vi "Build Filename.vi"(9 "Measurment Type":string, 11 "Metadata In":string[][](array[string])) -> (3 "String":string)   [LabVIEW 2014, in "Timing and Stabilization.lvlib"]
uses:
  Timing and Stabilization.lvlib
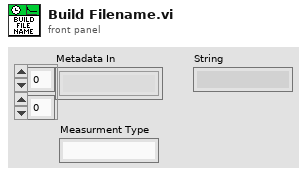
[diagram p1: front panel]
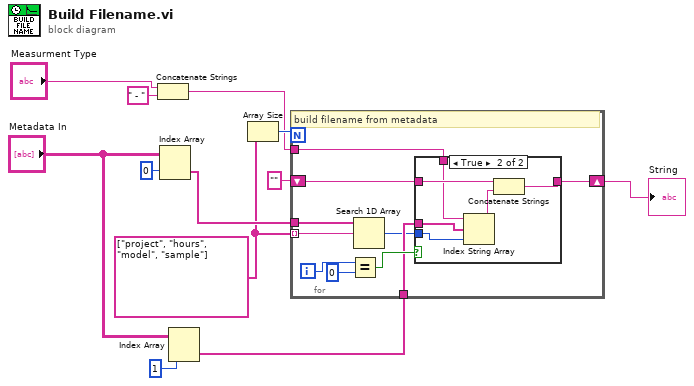
[diagram p0: block diagram]
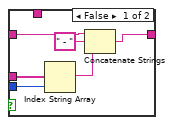
[diagram p2: hidden frame]
diagram:
  w7 = string[] ["project", "hours", "model", "sample"]
  n1 = Concatenate Strings("Measurment Type", " - " ("string")) -> (w3:string)
  n2 = Index Array(array="Metadata In", index (row)=0) -> (element=w10:string[])  [unwired: 1 in]
  n3 = Index Array(array="Metadata In", index (row)=1) -> (element=w11:string[])  [unwired: 1 in]
  n4 = Array Size(array=w7) -> (size(s)=w6:i32)
  n5 = for {
    N: w6 -> [_]
    tunnel: w10 -> [w16]
    shift-right: [w22] -> w5
    shift-left: "" -> [w21]
    tunnel: w7 -> [w17] mode=indexing
    tunnel: w11 -> [w15]
    tunnel: w3 -> [w13]
    i -> [w20]
    # "build filename from metadata"
    n6 = Equal?(x=w20, y=0) -> (x = y?=w18:bool)
    n7 = Search 1D Array(1D array=w16, element=w17) -> (index of element=w14:i32)  [unwired: 1 in]
    n8 = case shown="True" w18 {
      tunnel: [w27 w34] -> w22
      tunnel: w21 -> [w28 w33]
      tunnel: w15 -> [w24 w31]
      tunnel: w14 -> [w23 w30]
      tunnel: w13 -> [_ w29]
      frame False {
        n9 = Index String Array(1:w23, 2:w24) -> (0:w25:string)  [unwired: 1 in]
        n10 = Concatenate Strings(w28, " - " ("string"), w25) -> (w27:string)
      }
      frame True {
        n11 = Index String Array(1:w30, 2:w31, 3:w29) -> (0:w32:string)
        n12 = Concatenate Strings(w33, w32) -> (w34:string)
      }
    }
  }
  "String" <- w5
